vi "Check Client Compression Change.vi"(11 "Video Compression":refnum<vi>) -> ()   [LabVIEW 2023]
uses:
  <vilib>/Rock Robotics/Network Tables/NT Read Integer.vi
  <vilib>/Rock Robotics/Network Tables/NT Write Integer.vi
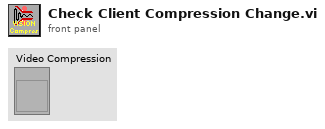
[diagram p1: front panel]
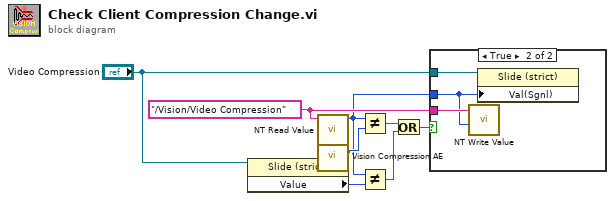
[diagram p0: block diagram]
diagram:
  w8 = "/Vision/Video Compression" ("Name")
  n1 = property class="Slide (strict)"(reference="Video Compression") -> ("Value"=w4:i32)  [unwired: 1 in, 2 out]
  n2 = call-poly <vilib>:"NT Read Value.vi"("name"=w8) -> ("value"=w5:i64)  [unwired: 8 in, 2 out]
  n3 = call "Vision Compression AE.vi"() -> ("Quality out"=w7:i32)  [unwired: 10 in, 1 out]
  n4 = Not Equal?(x=w5, y=w7) -> (x != y?=w2:bool)
  n5 = Not Equal?(x=w5, y=w4) -> (x != y?=w1:bool)
  n6 = Or(x=w2, y=w1) -> (x .or. y?=w3:bool)
  n7 = case shown="True" w3 {
    tunnel: w8 -> [_ w11]
    tunnel: "Video Compression" -> [_ w10]
    tunnel: w5 -> [_ w9]
    frame False {
    }
    frame True {
      n8 = call-poly <vilib>:"NT Write Value.vi"("value"=w9, "name"=w11) -> ()  [unwired: 9 in, 1 out]
      n9 = property class="Slide (strict)"(reference=w10, "Val(Sgnl)"=w9) -> ()  [unwired: 1 in, 2 out]
    }
  }
